vi "axis to can.vi"(5 "send speed over can":T1, 6 "ROS":bool, 7 "wej auto":T2 {"zadany" format="%<%H:%M:%S\n%x>T"}, 8 "wej ster":cluster{"Y axis":dbl, "X axis":dbl}, 9 "wej  ID":T5={"STM Lewy ID 1"=2, "STM Prawy ID 2"=1, "IDD 1"=1, "IDD 2"=1}, 10 "wej wagi":T4, 11 "ROS in":cluster{dbl, dbl}) -> (0 "array of cans":T6[](array[typedef]) {"type" items=["CAN Data", "CAN Remote"]; "identifier" format="%.0x"}, 2 "wyj pred":cluster{i16, i16, i16, i16, i16, i16} {"?" scale=-32767.0..32767.0; "?" scale=-32767.0..32767.0; "?" scale=-32767.0..32767.0; "?" scale=-32767.0..32767.0; "?" scale=-32767.0..32767.0; "?" scale=-32767.0..32767.0}, 3 "wyj auto":T3, 4 "wyœlij":bool=TRUE)   [LabVIEW 2015]
uses:
  CANFrameControl.ctl
  PC/wyj auto.ctl
panel:
  in  "reset":bool
  out "Time has Elapsed":bool
  out "Elapsed Time (s)":dbl
  out "zadany czas":bool
  out "AUTO ?":bool
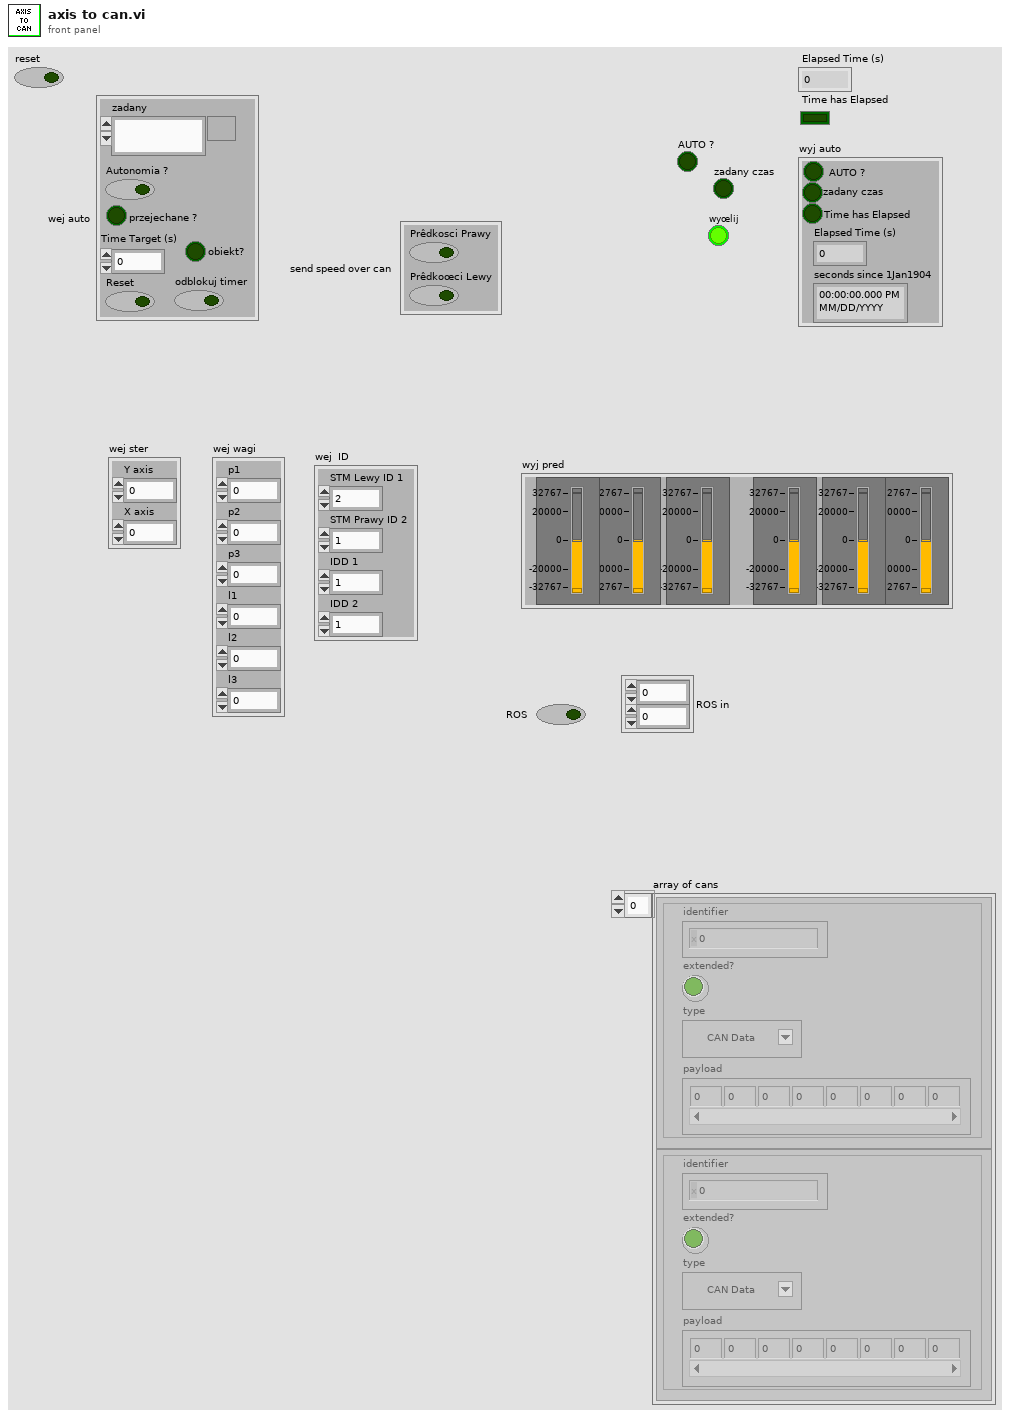
[diagram p1: front panel]
types:
  T1 = cluster{"Prêdkosci Prawy":bool, "Prêdkoœci Lewy":bool}
  T2 = cluster{"zadany":timestamp, "Autonomia ?":bool, "Time Target (s)":dbl, "Reset":bool, "odblokuj timer":bool, "obiekt?":bool, "przejechane ? ":bool}
  T3 = typedef "wyj auto.ctl" = cluster{"AUTO ?":bool, "zadany czas":bool, "Time has Elapsed":bool, "Elapsed Time (s)":dbl, "seconds since 1Jan1904":timestamp}
  T4 = cluster{"p1":dbl, "p2":dbl, "p3":dbl, "l1":dbl, "l2":dbl, "l3":dbl}
  T5 = cluster{"STM Lewy ID 1":u32, "STM Prawy ID 2":u32, "IDD 1":u8, "IDD 2":u8}
  T6 = typedef "CANFrameControl.ctl" = cluster{"identifier":u32, "extended?":bool, "type":u8, "payload":u8[]}
  T7 = cluster{bool, bool, "Time has Elapsed":bool, "Elapsed Time (s)":dbl, "seconds since 1Jan1904":timestamp}
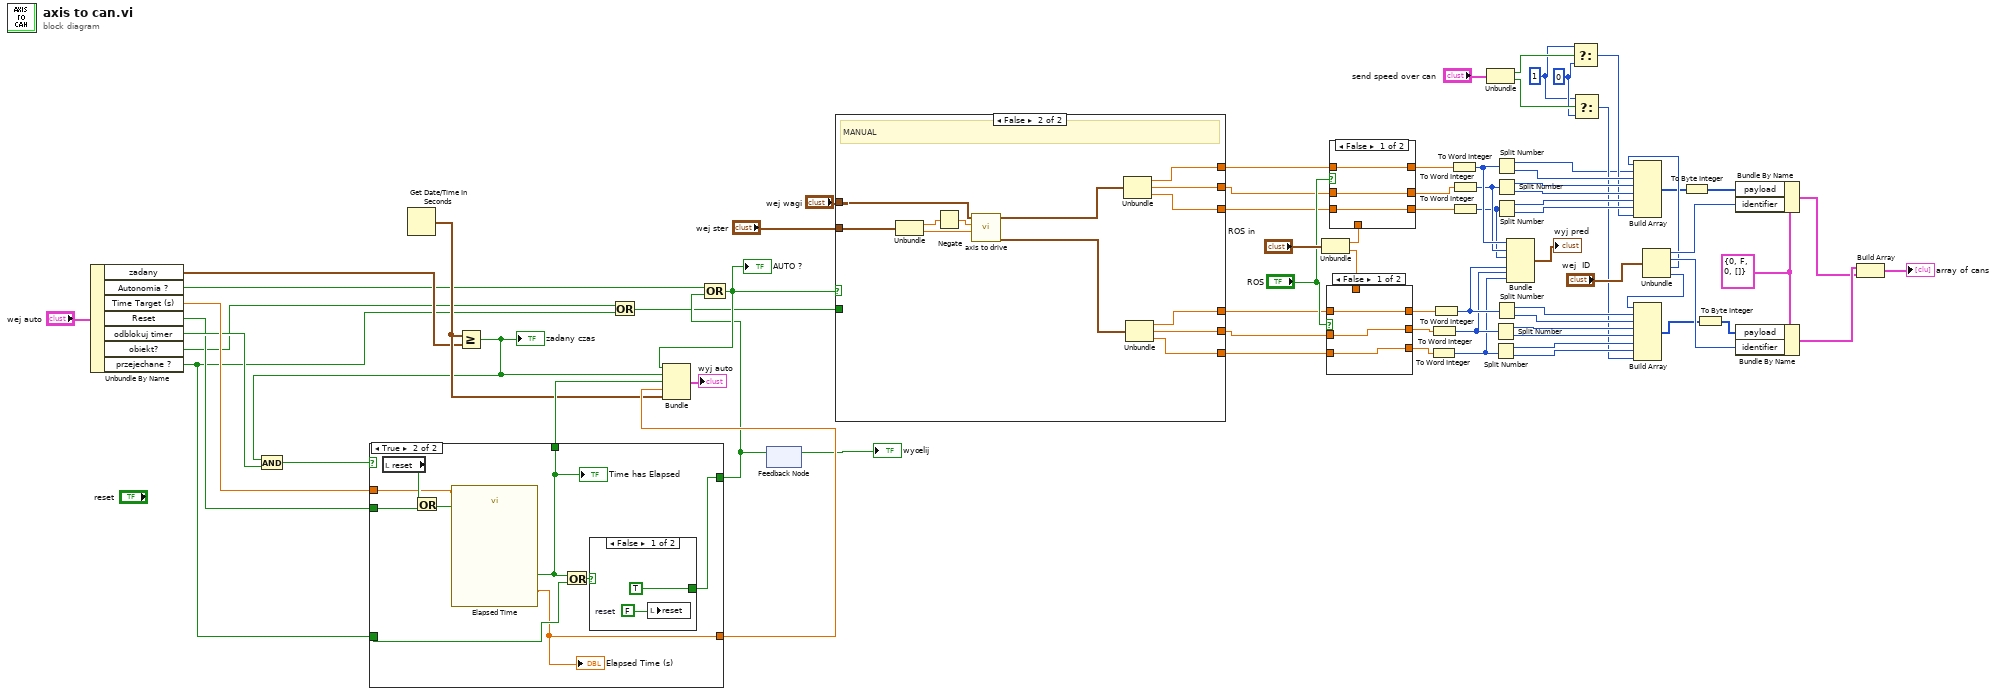
[diagram p0: block diagram]
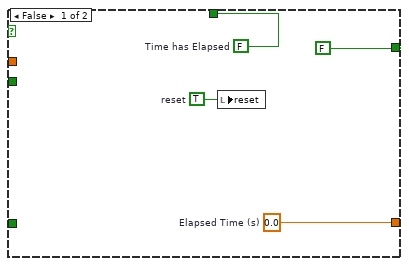
[diagram p4: hidden frame]
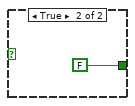
[diagram p5: hidden frame]
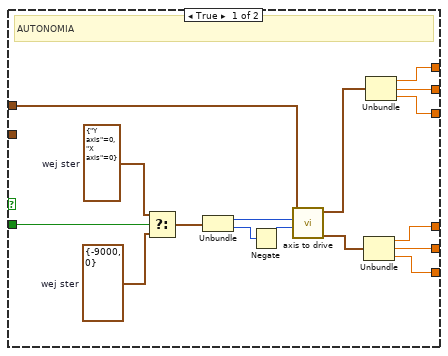
[diagram p6: hidden frame]
diagram:
  w22 = u8 1 ("element")
  w23 = u8 0 ("element")
  w75 = T6 {"identifier"=0, "extended?"=FALSE, "type"=0, "payload"=[]} ("CAN frame 2")
  n1 = Unbundle By Name("wej auto") -> ("zadany"=w41:timestamp, "Autonomia ?"=w36:bool, "Time Target (s)"=w43:dbl, "Reset"=w34:bool, "odblokuj timer"=w38:bool, "obiekt?"=w31:bool, "przejechane ?"=w29:bool)
  n2 = Get Date/Time In Seconds() -> (seconds since 1Jan1904=w42:timestamp)
  n3 = Greater Or Equal?(x=w42, y=w41) -> (x >= y?=w39:bool)
  "zadany czas" <- w39
  n4 = And(x=w39, y=w38) -> (x .and. y?=w40:bool)
  n5 = case shown="True" w40 {
    tunnel: [FALSE w88] -> w35
    tunnel: [w77 w81] -> w46
    tunnel: [w78 w80] -> w45
    tunnel: w34 -> [_ w87]
    tunnel: w43 -> [_ w82]
    tunnel: w29 -> [_ w84]
    frame False {
      w76 = TRUE  # reset
      w78 = 0.0  # Elapsed Time (s)
      w77 = FALSE  # Time has Elapsed
      n6 = local write "reset"(w76) -> ()
    }
    frame True {
      n7 = local read "reset"() -> (w86:bool)
      n8 = Or(x=w86, y=w87) -> (x .or. y?=w83:bool)
      n9 = call "Elapsed Time"("Time Target (s)"=w82, "Reset"=w83) -> ("Elapsed Time (s)"=w80:dbl, "Time has Elapsed"=w81:bool)  [unwired: 10 in, 6 out]
      "Elapsed Time (s)" <- w80
      "Time has Elapsed" <- w81
      n10 = Or(x=w81, y=w84) -> (x .or. y?=w85:bool)
      n11 = case shown="False" w85 {
        tunnel: [TRUE FALSE] -> w88
        frame False {
          w89 = FALSE  # reset
          n12 = local write "reset"(w89) -> ()
        }
        frame True {
        }
      }
    }
  }
  n13 = Or(x=w31, y=w29) -> (x .or. y?=w30:bool)
  n14 = Compound Arithmetic op=OR(w36, w35) -> (w37:bool)
  "AUTO ?" <- w37
  n15 = Bundle(w37, w39, "Time has Elapsed"=w46, "Elapsed Time (s)"=w45, "seconds since 1Jan1904"=w42) -> (→"wyj auto":T7)  [unwired: 1 in]
  n16 = feedback-in #1(w35) -> ()
  n17 = feedback #1() -> (→"wyœlij":bool)  [unwired: 1 in]
  n18 = case shown="False" w37 {
    tunnel: [w96 w112] -> w12
    tunnel: [w95 w113] -> w10
    tunnel: [w94 w111] -> w8
    tunnel: [w97 w115] -> w14
    tunnel: [w98 w116] -> w17
    tunnel: [w99 w117] -> w19
    tunnel: "wej ster" -> [_ w120]
    tunnel: "wej wagi" -> [w104 w119]
    tunnel: w30 -> [w92 _]
    frame True {
      w102 = cluster{"Y axis":i32, "X axis":i32} {"Y axis"=0, "X axis"=0}  # wej ster
      w101 = cluster{"Y axis":i32, "X axis":i32} {"Y axis"=-9000, "X axis"=0}  # wej ster
      # "AUTONOMIA"
      n19 = Select(t=w102, s=w92, f=w101) -> (s? t:f=w103:cluster{"Y axis":i32, "X axis":i32})
      n20 = Unbundle(w103) -> ("Y axis"=w105:i32, "X axis"=w107:i32)
      n21 = Negate(x=w107) -> (-x=w106:i32)
      n22 = call "axis to drive.vi"("X axis"=w106, "Y axis"=w105, "wej wagi"=w104) -> ("wyj P"=w93:cluster{"y":dbl, "y":dbl, "y":dbl}, "wyj L"=w100:cluster{"y":dbl, "y":dbl, "y":dbl})  [unwired: 7 in]
      n23 = Unbundle(w93) -> ("y"=w96:dbl, "y"=w95:dbl, "y"=w94:dbl)
      n24 = Unbundle(w100) -> ("y"=w99:dbl, "y"=w98:dbl, "y"=w97:dbl)
    }
    frame False {
      # "MANUAL"
      n25 = Unbundle(w120) -> ("Y axis"=w109:dbl, "X axis"=w110:dbl)
      n26 = Negate(x=w109) -> (-x=w108:dbl)
      n27 = call "axis to drive.vi"("X axis"=w110, "Y axis"=w108, "wej wagi"=w119) -> ("wyj P"=w114:cluster{"y":dbl, "y":dbl, "y":dbl}, "wyj L"=w118:cluster{"y":dbl, "y":dbl, "y":dbl})  [unwired: 7 in]
      n28 = Unbundle(w118) -> ("y"=w117:dbl, "y"=w116:dbl, "y"=w115:dbl)
      n29 = Unbundle(w114) -> ("y"=w112:dbl, "y"=w113:dbl, "y"=w111:dbl)
    }
  }
  n30 = Unbundle("ROS in") -> (w7:dbl, w6:dbl)
  n31 = case shown="False" "ROS" {
    tunnel: [w123 w124] -> w13
    tunnel: w12 -> [w123 _]
    tunnel: [w122 w124] -> w11
    tunnel: w10 -> [w122 _]
    tunnel: [w121 w124] -> w9
    tunnel: w8 -> [w121 _]
    tunnel: w6 -> [_ w124]
    frame False {
    }
    frame True {
    }
  }
  n32 = case shown="False" "ROS" {
    tunnel: w19 -> [w126 _]
    tunnel: [w127 w128] -> w18
    tunnel: w17 -> [w127 _]
    tunnel: [w126 w128] -> w16
    tunnel: [w125 w128] -> w15
    tunnel: w14 -> [w125 _]
    tunnel: w7 -> [_ w128]
    frame False {
    }
    frame True {
    }
  }
  n33 = To Word Integer(number=w9) -> (16bit integer=w50:i16)
  n34 = To Word Integer(number=w11) -> (16bit integer=w51:i16)
  n35 = To Word Integer(number=w13) -> (16bit integer=w52:i16)
  n36 = To Word Integer(number=w16) -> (16bit integer=w55:i16)
  n37 = To Word Integer(number=w18) -> (16bit integer=w54:i16)
  n38 = To Word Integer(number=w15) -> (16bit integer=w53:i16)
  n39 = Unbundle("send speed over can") -> ("Prêdkosci Prawy"=w27:bool, "Prêdkoœci Lewy"=w26:bool)
  n40 = Split Number(x=w51) -> (hi(x)=w64:u8, lo(x)=w63:u8)
  n41 = Split Number(x=w50) -> (hi(x)=w62:u8, lo(x)=w61:u8)
  n42 = Split Number(x=w55) -> (hi(x)=w5:u8, lo(x)=w71:u8)
  n43 = Split Number(x=w54) -> (hi(x)=w68:u8, lo(x)=w67:u8)
  n44 = Split Number(x=w53) -> (hi(x)=w66:u8, lo(x)=w65:u8)
  n45 = Split Number(x=w52) -> (hi(x)=w70:u8, lo(x)=w69:u8)
  n46 = Bundle(w55, w54, w53, w52, w51, w50) -> (→"wyj pred":cluster{i16, i16, i16, i16, i16, i16})  [unwired: 1 in]
  n47 = Select(t=w22, s=w27, f=w23) -> (s? t:f=w25:u8)
  n48 = Select(t=w22, s=w26, f=w23) -> (s? t:f=w24:u8)
  n49 = Unbundle("wej  ID") -> ("STM Lewy ID 1"=w59:u32, "STM Prawy ID 2"=w58:u32, "IDD 1"=w57:u8, "IDD 2"=w56:u8)
  n50 = Build Array(w57, w5, w71, w68, w67, w66, w65, w25) -> (w3:u8[])
  n51 = Build Array(w56, w70, w69, w64, w63, w62, w61, w24) -> (w1:u8[])
  n52 = To Byte Integer(number=w3) -> (8bit integer=w4:i8[])
  n53 = To Byte Integer(number=w1) -> (8bit integer=w2:i8[])
  n54 = Bundle By Name(cluster=w75, "payload"=w4, "identifier"=w59) -> (w73:T6)
  n55 = Bundle By Name(cluster=w75, "payload"=w2, "identifier"=w58) -> (w74:T6)
  n56 = Build Array(w74, w73) -> (→"array of cans":T6[])
